vi "Get Status.vi"(8 "error in (no error)":errorcluster, 11 "GaGe Digitizer in":refnum<class "GaGe Digitizer.lvclass">) -> (0 "error out":errorcluster, 2 "Complete":bool, 3 "GaGe Digitizer out":refnum<class "GaGe Digitizer.lvclass">, 4 "Triggered":bool, 5 "Armed":bool)   [LabVIEW 2015, in "GaGe Digitizer.lvclass"]
uses:
  GaGe Digitizer.lvclass
  GaGe Digitizer.lvclass/GaGe Digitizer.ctl
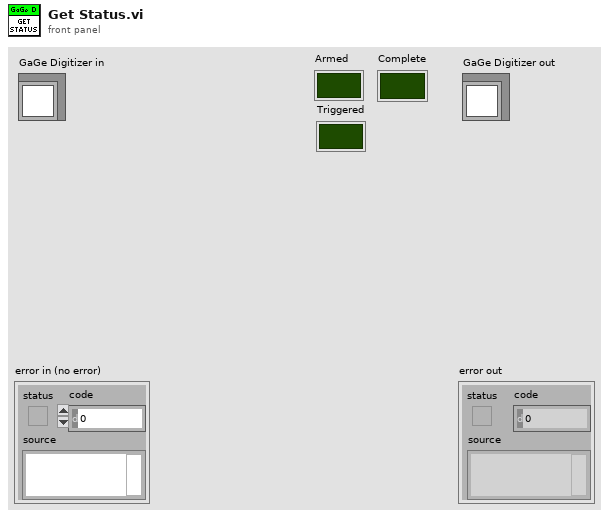
[diagram p1: front panel]
types:
  T1 = cluster{"Handle":u32, "Sample size":u32, "Resolution":i32, "Offset":i32, "Channels":u32, "Boards":u32}
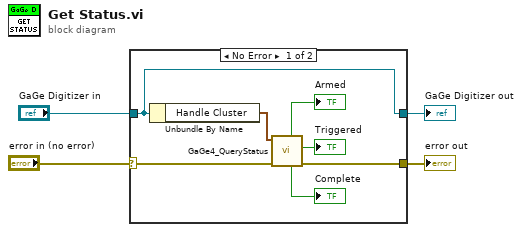
[diagram p0: block diagram]
diagram:
  n1 = case shown="No Error" "error in (no error)" {
    selector: "error in (no error)" -> [w7 w13]
    tunnel: [w6 w13] -> w3
    tunnel: [w11 w12] -> w1
    tunnel: "GaGe Digitizer in" -> [w11 w12]
    frame No Error {
      n2 = Unbundle By Name(w11) -> ("Handle Cluster"=w10:T1)
      n3 = call "GaGe4_QueryStatus.vi"("error in (no error)"=w7, "Handle Cluster"=w10) -> ("error out"=w6:errorcluster, "Triggered"=→"Triggered":bool, "Complete"=→"Complete":bool, "Armed"=→"Armed":bool)  [unwired: 4 in, 2 out]
    }
    frame Error {
    }
  }
  "error out" <- w3
  "GaGe Digitizer out" <- w1
